vi "nanocal -- nuclear schottky fit V7.vi"() -> ()   [LabVIEW 2021] (continued)
,  \"στ1\" -> 0.000000000000   ,  \"στS\" -> 0.000000000000   ,  \"στN\" -> 0.000000000000    |>   , \n\"IDS0213_210310_RAW_cal__ref_\" ->   <|    \"ζ\" -> 0.158514180755   ,  \"τ1\" -> 0.046388884826   ,  \"τS\" -> 0.038847986012   ,  \"τN\" -> 0.058494864948   ,  \"τC\" -> 0.001325817289   ,  \"κ0\" -> 0.000000001072   ,  \"mm1\" -> 0.000176864175   ,  \"mm2\" -> 0.014706895751   ,  \"mm3\" -> 0.145604015421   ,  \"T\" -> 0.197000000000   ,  \"B\" -> 10.000000000000   ,  \"θ\" -> 0.000000000000   ,  \"Reoff\" -> 0.000000000000   ,  \"Imoff\" -> 0.000000000000   ,  \"στ1\" -> 0.000000000000   ,  \"στS\" -> 0.000000000000   ,  \"στN\" -> 0.000000000000    |>   , \n\"IDS0213_210310_RAW_cal__sam_\" ->   <|    \"ζ\" -> 0.130083148284   ,  \"τ1\" -> 0.046211117525   ,  \"τS\" -> 0.046173592526   ,  \"τN\" -> 0.081942172735   ,  \"τC\" -> 0.001380184863   ,  \"κ0\" -> 0.000000001209   ,  \"mm1\" -> 0.000155206642   ,  \"mm2\" -> 0.013836953800   ,  \"mm3\" -> 0.178380609297   ,  \"T\" -> 0.197000000000   ,  \"B\" -> 10.000000000000   ,  \"θ\" -> 0.000000000000   ,  \"Reoff\" -> 0.000000000000   ,  \"Imoff\" -> 0.000000000000   ,  \"στ1\" -> 0.000000000000   ,  \"στS\" -> 0.000000000000   ,  \"στN\" -> 0.000000000000    |>   , \n\"IDS0214_210310_RAW_cal__ref_\" ->   <|    \"ζ\" -> 0.154362032240   ,  \"τ1\" -> 0.030258273194   ,  \"τS\" -> 0.049523350330   ,  \"τN\" -> 0.040015703513   ,  \"τC\" -> 0.001328953616   ,  \"κ0\" -> 0.000000001075   ,  \"mm1\" -> 0.000174173720   ,  \"mm2\" -> 0.014698349376   ,  \"mm3\" -> 0.120075187874   ,  \"T\" -> 0.197000000000   ,  \"B\" -> 8.000000000000   ,  \"θ\" -> 0.000000000000   ,  \"Reoff\" -> 0.000000000000   ,  \"Imoff\" -> 0.000000000000   ,  \"στ1\" -> 0.000000000000   ,  \"στS\" -> 0.000000000000   ,  \"στN\" -> 0.000000000000    |>   , \n\"IDS0214_210310_RAW_cal__sam_\" ->   <|    \"ζ\" -> 0.126440702434   ,  \"τ1\" -> 0.034118036572   ,  \"τS\" -> 0.060921114440   ,  \"τN\" -> 0.059832148427   ,  \"τC\" -> 0.001404471084   ,  \"κ0\" -> 0.000000001199   ,  \"mm1\" -> 0.000154817132   ,  \"mm2\" -> 0.015271462818   ,  \"mm3\" -> 0.156117617951   ,  \"T\" -> 0.197000000000   ,  \"B\" -> 8.000000000000   ,  \"θ\" -> 0.000000000000   ,  \"Reoff\" -> 0.000000000000   ,  \"Imoff\" -> 0.000000000000   ,  \"στ1\" -> 0.000000000000   ,  \"στS\" -> 0.000000000000   ,  \"στN\" -> 0.000000000000    |>   , \n\"IDS0215_210310_RAW_cal__ref_\" ->   <|    \"ζ\" -> 0.162645417184   ,  \"τ1\" -> 0.023693851446   ,  \"τS\" -> 0.062400062170   ,  \"τN\" -> 0.026326088223   ,  \"τC\" -> 0.001322053294   ,  \"κ0\" -> 0.000000001070   ,  \"mm1\" -> 0.000182075033   ,  \"mm2\" -> 0.015525359924   ,  \"mm3\" -> 0.112465521923   ,  \"T\" -> 0.197000000000   ,  \"B\" -> 7.000000000000   ,  \"θ\" -> 0.000000000000   ,  \"Reoff\" -> 0.000000000000   ,  \"Imoff\" -> 0.000000000000   ,  \"στ1\" -> 0.000000000000   ,  \"στS\" -> 0.000000000000   ,  \"στN\" -> 0.000000000000    |>   , \n\"IDS0215_210310_RAW_cal__sam_\" ->   <|    \"ζ\" -> 0.131383255045   ,  \"τ1\" -> 0.026827335842   ,  \"τS\" -> 0.071725959535   ,  \"τN\" -> 0.047510049318   ,  \"τC\" -> 0.001407613780   ,  \"κ0\" -> 0.000000001187   ,  \"mm1\" -> 0.000160977956   ,  \"mm2\" -> 0.014932130994   ,  \"mm3\" -> 0.148043464486   ,  \"T\" -> 0.197000000000   ,  \"B\" -> 7.000000000000   ,  \"θ\" -> 0.000000000000   ,  \"Reoff\" -> 0.000000000000   ,  \"Imoff\" -> 0.000000000000   ,  \"στ1\" -> 0.000000000000   ,  \"στS\" -> 0.000000000000   ,  \"στN\" -> 0.000000000000    |>   , \n\"IDS0216_210310_RAW_cal__ref_\" ->   <|    \"ζ\" -> 0.149904026692   ,  \"τ1\" -> 0.020347243982   ,  \"τS\" -> 0.075273674904   ,  \"τN\" -> 0.020640082408   ,  \"τC\" -> 0.001432916876   ,  \"κ0\" -> 0.000000001050   ,  \"mm1\" -> 0.000184134986   ,  \"mm2\" -> 0.015328528282   ,  \"mm3\" -> 0.116559113338   ,  \"T\" -> 0.197000000000   ,  \"B\" -> 5.000000000000   ,  \"θ\" -> 0.000000000000   ,  \"Reoff\" -> 0.000000000000   ,  \"Imoff\" -> 0.000000000000   ,  \"στ1\" -> 0.000000000000   ,  \"στS\" -> 0.000000000000   ,  \"στN\" -> 0.000000000000    |>   , \n\"IDS0216_210310_RAW_cal__sam_\" ->   <|    \"ζ\" -> 0.125455081262   ,  \"τ1\" -> 0.021777951907   ,  \"τS\" -> 0.089086097551   ,  \"τN\" -> 0.033580911935   ,  \"τC\" -> 0.001437991682   ,  \"κ0\" -> 0.000000001167   ,  \"mm1\" -> 0.000158268021   ,  \"mm2\" -> 0.015150793318   ,  \"mm3\" -> 0.145963091379   ,  \"T\" -> 0.197000000000   ,  \"B\" -> 5.000000000000   ,  \"θ\" -> 0.000000000000   ,  \"Reoff\" -> 0.000000000000   ,  \"Imoff\" -> 0.000000000000   ,  \"στ1\" -> 0.000000000000   ,  \"στS\" -> 0.000000000000   ,  \"στN\" -> 0.000000000000    |>   , \n\"IDS0217_210310_RAW_cal__ref_\" ->   <|    \"ζ\" -> 0.121305227705   ,  \"τ1\" -> 0.032098202143   ,  \"τS\" -> 0.011865067519   ,  \"τN\" -> 0.005878702730   ,  \"τC\" -> 0.002147559783   ,  \"κ0\" -> 0.000000001032   ,  \"mm1\" -> 0.000202614262   ,  \"mm2\" -> 0.011552455211   ,  \"mm3\" -> 0.042386874792   ,  \"T\" -> 0.197000000000   ,  \"B\" -> 0.000000000000   ,  \"θ\" -> 0.000000000000   ,  \"Reoff\" -> 0.000000000000   ,  \"Imoff\" -> 0.000000000000   ,  \"στ1\" -> 0.000000000000   ,  \"στS\" -> 0.000000000000   ,  \"στN\" -> 0.000000000000    |>   , \n\"IDS0217_210310_RAW_cal__sam_\" ->   <|    \"ζ\" -> 0.101804363109   ,  \"τ1\" -> 0.031947692776   ,  \"τS\" -> 0.014125667853   ,  \"τN\" -> 0.006009042128   ,  \"τC\" -> 0.002323789932   ,  \"κ0\" -> 0.000000001168   ,  \"mm1\" -> 0.000188754224   ,  \"mm2\" -> 0.013103876414   ,  \"mm3\" -> 0.043163363377   ,  \"T\" -> 0.197000000000   ,  \"B\" -> 0.000000000000   ,  \"θ\" -> 0.000000000000   ,  \"Reoff\" -> 0.000000000000   ,  \"Imoff\" -> 0.000000000000   ,  \"στ1\" -> 0.000000000000   ,  \"στS\" -> 0.000000000000   ,  \"στN\" -> 0.000000000000    |>   , \n\"IDS0218_210310_RAW_cal__ref_\" ->   <|    \"ζ\" -> 0.000000000000   ,  \"τ1\" -> 0.000000000000   ,  \"τS\" -> 0.000000000000   ,  \"τN\" -> 0.000000000000   ,  \"τC\" -> 0.000000000000   ,  \"κ0\" -> 0.000000000000   ,  \"mm1\" -> 0.000000000000   ,  \"mm2\" -> 0.000000000000   ,  \"mm3\" -> 0.000000000000   ,  \"T\" -> 1.550000000000   ,  \"B\" -> 0.000000000000   ,  \"θ\" -> 0.000000000000   ,  \"Reoff\" -> 0.000000000000   ,  \"Imoff\" -> 0.000000000000   ,  \"στ1\" -> 0.000000000000   ,  \"στS\" -> 0.000000000000   ,  \"στN\" -> 0.000000000000    |>   , \n\"IDS0218_210310_RAW_cal__sam_\" ->   <|    \"ζ\" -> 0.008537038929   ,  \"τ1\" -> 0.006154643814   ,  \"τS\" -> 0.040521205127   ,  \"τN\" -> 0.000711776675   ,  \"τC\" -> 0.001925410383   ,  \"κ0\" -> 0.000000011800   ,  \"mm1\" -> 0.000015570479   ,  \"mm2\" -> 0.006036709260   ,  \"mm3\" -> 0.043612763831   ,  \"T\" -> 1.550000000000   ,  \"B\" -> 0.000000000000   ,  \"θ\" -> 0.000000000000   ,  \"Reoff\" -> -420408.163265306153   ,  \"Imoff\" -> 0.000000000000   ,  \"στ1\" -> 0.000216261088   ,  \"στS\" -> 0.000541561495   ,  \"στN\" -> 0.000022390164    |>   , \n\"IDS0219_210310_RAW_cal__ref_\" ->   <|    \"ζ\" -> 0.000000000000   ,  \"τ1\" -> 0.000000000000   ,  \"τS\" -> 0.000000000000   ,  \"τN\" -> 0.000000000000   ,  \"τC\" -> 0.000000000000   ,  \"κ0\" -> 0.000000000000   ,  \"mm1\" -> 0.000000000000   ,  \"mm2\" -> 0.000000000000   ,  \"mm3\" -> 0.000000000000   ,  \"T\" -> 1.000000000000   ,  \"B\" -> 0.000000000000   ,  \"θ\" -> 0.000000000000   ,  \"Reoff\" -> 0.000000000000   ,  \"Imoff\" -> 0.000000000000   ,  \"στ1\" -> 0.000000000000   ,  \"στS\" -> 0.000000000000   ,  \"στN\" -> 0.000000000000    |>   , \n\"IDS0219_210310_RAW_cal__sam_\" ->   <|    \"ζ\" -> 0.000000000000   ,  \"τ1\" -> 0.000000000000   ,  \"τS\" -> 0.000000000000   ,  \"τN\" -> 0.000000000000   ,  \"τC\" -> 0.000000000000   ,  \"κ0\" -> 0.000000000000   ,  \"mm1\" -> 0.000000000000   ,  \"mm2\" -> 0.000000000000   ,  \"mm3\" -> 0.000000000000   ,  \"T\" -> 1.000000000000   ,  \"B\" -> 0.000000000000   ,  \"θ\" -> 0.000000000000   ,  \"Reoff\" -> 0.000000000000   ,  \"Imoff\" -> 0.000000000000   ,  \"στ1\" -> 0.000000000000   ,  \"στS\" -> 0.000000000000   ,  \"στN\" -> 0.000000000000    |>   , \n\"IDS0220_210310_RAW_cal__ref_\" ->   <|    \"ζ\" -> 0.000000000000   ,  \"τ1\" -> 0.000000000000   ,  \"τS\" -> 0.000000000000   ,  \"τN\" -> 0.000000000000   ,  \"τC\" -> 0.000000000000   ,  \"κ0\" -> 0.000000000000   ,  \"mm1\" -> 0.000000000000   ,  \"mm2\" -> 0.000000000000   ,  \"mm3\" -> 0.000000000000   ,  \"T\" -> 0.677000000000   ,  \"B\" -> 0.000000000000   ,  \"θ\" -> 0.000000000000   ,  \"Reoff\" -> 0.000000000000   ,  \"Imoff\" -> 0.000000000000   ,  \"στ1\" -> 0.000000000000   ,  \"στS\" -> 0.000000000000   ,  \"στN\" -> 0.000000000000    |>   , \n\"IDS0220_210310_RAW_cal__sam_\" ->   <|    \"ζ\" -> 0.000000000000   ,  \"τ1\" -> 0.000000000000   ,  \"τS\" -> 0.000000000000   ,  \"τN\" -> 0.000000000000   ,  \"τC\" -> 0.000000000000   ,  \"κ0\" -> 0.000000000000   ,  \"mm1\" -> 0.000000000000   ,  \"mm2\" -> 0.000000000000   ,  \"mm3\" -> 0.000000000000   ,  \"T\" -> 0.677000000000   ,  \"B\" -> 0.000000000000   ,  \"θ\" -> 0.000000000000   ,  \"Reoff\" -> 0.000000000000   ,  \"Imoff\" -> 0.000000000000   ,  \"στ1\" -> 0.000000000000   ,  \"στS\" -> 0.000000000000   ,  \"στN\" -> 0.000000000000    |>   , \n\"IDS0224_210310_RAW_cal__ref_\" ->   <|    \"ζ\" -> 0.000000000000   ,  \"τ1\" -> 0.000000000000   ,  \"τS\" -> 0.000000000000   ,  \"τN\" -> 0.000000000000   ,  \"τC\" -> 0.000000000000   ,  \"κ0\" -> 0.000000000000   ,  \"mm1\" -> 0.000000000000   ,  \"mm2\" -> 0.000000000000   ,  \"mm3\" -> 0.000000000000   ,  \"T\" -> 0.000000000000   ,  \"B\" -> 0.000000000000   ,  \"θ\" -> 0.000000000000   ,  \"Reoff\" -> 0.000000000000   ,  \"Imoff\" -> 0.000000000000   ,  \"στ1\" -> 0.000000000000   ,  \"στS\" -> 0.000000000000   ,  \"στN\" -> 0.000000000000    |>   , \n\"IDS0224_210310_RAW_cal__sam_\" ->   <|    \"ζ\" -> 0.000000000000   ,  \"τ1\" -> 0.000000000000   ,  \"τS\" -> 0.000000000000   ,  \"τN\" -> 0.000000000000   ,  \"τC\" -> 0.000000000000   ,  \"κ0\" -> 0.000000000000   ,  \"mm1\" -> 0.000000000000   ,  \"mm2\" -> 0.000000000000   ,  \"mm3\" -> 0.000000000000   ,  \"T\" -> 0.000000000000   ,  \"B\" -> 0.000000000000   ,  \"θ\" -> 0.000000000000   ,  \"Reoff\" -> 0.000000000000   ,  \"Imoff\" -> 0.000000000000   ,  \"στ1\" -> 0.000000000000   ,  \"στS\" -> 0.000000000000   ,  \"στN\" -> 0.000000000000    |>   , \n\"IDS0293_210427_RAW_cal__ref_\" ->   <|    \"ζ\" -> 0.016384838586   ,  \"τ1\" -> 0.013784349529   ,  \"τS\" -> 0.011495286759   ,  \"τN\" -> 0.000117117954   ,  \"τC\" -> 0.004048153799   ,  \"κ0\" -> 0.000000013122   ,  \"mm1\" -> 0.000048616206   ,  \"mm2\" -> 0.013163310838   ,  \"mm3\" -> 0.016423248374   ,  \"T\" -> 1.900000000000   ,  \"B\" -> 12.000000000000   ,  \"θ\" -> 30.000000000000   ,  \"Reoff\" -> 0.000000000000   ,  \"Imoff\" -> 0.000000000000   ,  \"στ1\" -> 0.000000000000   ,  \"στS\" -> 0.000000000000   ,  \"στN\" -> 0.000000000000    |>   , \n\"IDS0293_210427_RAW_cal__sam_\" ->   <|    \"ζ\" -> 0.009769235649   ,  \"τ1\" -> 0.020538276815   ,  \"τS\" -> 0.013494754544   ,  \"τN\" -> 0.000177075548   ,  \"τC\" -> 0.005872879859   ,  \"κ0\" -> 0.000000013933   ,  \"mm1\" -> 0.000039786676   ,  \"mm2\" -> 0.018120715591   ,  \"mm3\" -> 0.022056047829   ,  \"T\" -> 1.900000000000   ,  \"B\" -> 12.000000000000   ,  \"θ\" -> 30.000000000000   ,  \"Reoff\" -> -172000.000000000000   ,  \"Imoff\" -> 0.000000000000   ,  \"στ1\" -> 0.000000000000   ,  \"στS\" -> 0.000000000000   ,  \"στN\" -> 0.000000000000    |>   , \n\"IDS0294_210427_RAW_cal__ref_\" ->   <|    \"ζ\" -> 0.017975147456   ,  \"τ1\" -> 0.015573317032   ,  \"τS\" -> 0.016697357463   ,  \"τN\" -> 0.000401487663   ,  \"τC\" -> 0.004243374884   ,  \"κ0\" -> 0.000000007622   ,  \"mm1\" -> 0.000060128790   ,  \"mm2\" -> 0.014656172673   ,  \"mm3\" -> 0.022506589842   ,  \"T\" -> 1.130000000000   ,  \"B\" -> 12.000000000000   ,  \"θ\" -> 30.000000000000   ,  \"Reoff\" -> 0.000000000000   ,  \"Imoff\" -> 0.000000000000   ,  \"στ1\" -> 0.000000000000   ,  \"στS\" -> 0.000000000000   ,  \"στN\" -> 0.000000000000    |>   , \n\"IDS0294_210427_RAW_cal__sam_\" ->   <|    \"ζ\" -> 0.010952304636   ,  \"τ1\" -> 0.020329649306   ,  \"τS\" -> 0.020621176960   ,  \"τN\" -> 0.000487558003   ,  \"τC\" -> 0.005477732780   ,  \"κ0\" -> 0.000000008194   ,  \"mm1\" -> 0.000047079068   ,  \"mm2\" -> 0.019035053021   ,  \"mm3\" -> 0.028065174256   ,  \"T\" -> 1.130000000000   ,  \"B\" -> 12.000000000000   ,  \"θ\" -> 30.000000000000   ,  \"Reoff\" -> -250000.000000000000   ,  \"Imoff\" -> 0.000000000000   ,  \"στ1\" -> 0.000000000000   ,  \"στS\" -> 0.000000000000   ,  \"στN\" -> 0.000000000000    |>   , \n\"IDS0295_210427_RAW_cal__ref_\" ->   <|    \"ζ\" -> 0.021360373560   ,  \"τ1\" -> 0.017226807214   ,  \"τS\" -> 0.021136224671   ,  \"τN\" -> 0.000857882935   ,  \"τC\" -> 0.004088468956   ,  \"κ0\" -> 0.000000005432   ,  \"mm1\" -> 0.000072090186   ,  \"mm2\" -> 0.015812919970   ,  \"mm3\" -> 0.027894175974   ,  \"T\" -> 0.830000000000   ,  \"B\" -> 12.000000000000   ,  \"θ\" -> 30.000000000000   ,  \"Reoff\" -> 0.000000000000   ,  \"Imoff\" -> 0.000000000000   ,  \"στ1\" -> 0.000000000000   ,  \"στS\" -> 0.000000000000   ,  \"στN\" -> 0.000000000000    |>   , \n\"IDS0295_210427_RAW_cal__sam_\" ->   <|    \"ζ\" -> 0.014046811833   ,  \"τ1\" -> 0.021205417259   ,  \"τS\" -> 0.025982453768   ,  \"τN\" -> 0.000985536826   ,  \"τC\" -> 0.005692013080   ,  \"κ0\" -> 0.000000005890   ,  \"mm1\" -> 0.000064969808   ,  \"mm2\" -> 0.019619534974   ,  \"mm3\" -> 0.034559730440   ,  \"T\" -> 0.830000000000   ,  \"B\" -> 12.000000000000   ,  \"θ\" -> 30.000000000000   ,  \"Reoff\" -> -401999.999999999999   ,  \"Imoff\" -> 0.000000000000   ,  \"στ1\" -> 0.000000000000   ,  \"στS\" -> 0.000000000000   ,  \"στN\" -> 0.000000000000    |>   , \n\"IDS0296_210427_RAW_cal__ref_\" ->   <|    \"ζ\" -> 0.027756025784   ,  \"τ1\" -> 0.019742757718   ,  \"τS\" -> 0.026611973171   ,  \"τN\" -> 0.001398943183   ,  \"τC\" -> 0.003482574473   ,  \"κ0\" -> 0.000000003907   ,  \"mm1\" -> 0.000083653758   ,  \"mm2\" -> 0.017774350196   ,  \"mm3\" -> 0.034155716307   ,  \"T\" -> 0.620000000000   ,  \"B\" -> 12.000000000000   ,  \"θ\" -> 30.000000000000   ,  \"Reoff\" -> 0.000000000000   ,  \"Imoff\" -> 0.000000000000   ,  \"στ1\" -> 0.000000000000   ,  \"στS\" -> 0.000000000000   ,  \"στN\" -> 0.000000000000    |>   , \n\"IDS0296_210427_RAW_cal__sam_\" ->   <|    \"ζ\" -> 0.017388662959   ,  \"τ1\" -> 0.016835863979   ,  \"τS\" -> 0.033051741689   ,  \"τN\" -> 0.001876583642   ,  \"τC\" -> 0.004718731610   ,  \"κ0\" -> 0.000000004257   ,  \"mm1\" -> 0.000070854167   ,  \"mm2\" -> 0.015532685015   ,  \"mm3\" -> 0.041486738616   ,  \"T\" -> 0.620000000000   ,  \"B\" -> 12.000000000000   ,  \"θ\" -> 30.000000000000   ,  \"Reoff\" -> -602409.638554215430   ,  \"Imoff\" -> 0.000000000000   ,  \"στ1\" -> 0.000000000000   ,  \"στS\" -> 0.000000000000   ,  \"στN\" -> 0.000000000000    |>   , \n\"IDS0297_210427_RAW_cal__ref_\" ->   <|    \"ζ\" -> 0.034775017342   ,  \"τ1\" -> 0.018923965005   ,  \"τS\" -> 0.030086686370   ,  \"τN\" -> 0.002286572055   ,  \"τC\" -> 0.002714831651   ,  \"κ0\" -> 0.000000003294   ,  \"mm1\" -> 0.000084124720   ,  \"mm2\" -> 0.016628755460   ,  \"mm3\" -> 0.038424955523   ,  \"T\" -> 0.530000000000   ,  \"B\" -> 12.000000000000   ,  \"θ\" -> 30.000000000000   ,  \"Reoff\" -> 0.000000000000   ,  \"Imoff\" -> 0.000000000000   ,  \"στ1\" -> 0.000000000000   ,  \"στS\" -> 0.000000000000   ,  \"στN\" -> 0.000000000000    |>   , \n\"IDS0297_210427_RAW_cal__sam_\" ->   <|    \"ζ\" -> 0.020542184284   ,  \"τ1\" -> 0.020760439172   ,  \"τS\" -> 0.037341907366   ,  \"τN\" -> 0.003219016214   ,  \"τC\" -> 0.004292471555   ,  \"κ0\" -> 0.000000003557   ,  \"mm1\" -> 0.000077795275   ,  \"mm2\" -> 0.018267084885   ,  \"mm3\" -> 0.048102164115   ,  \"T\" -> 0.530000000000   ,  \"B\" -> 12.000000000000   ,  \"θ\" -> 30.000000000000   ,  \"Reoff\" -> -602409.638554215430   ,  \"Imoff\" -> 0.000000000000   ,  \"στ1\" -> 0.000000000000   ,  \"στS\" -> 0.000000000000   ,  \"στN\" -> 0.000000000000    |>   , \n\"IDS0298_210427_RAW_cal__ref_\" ->   <|    \"ζ\" -> 0.046440102993   ,  \"τ1\" -> 0.018907201785   ,  \"τS\" -> 0.034021724611   ,  \"τN\" -> 0.004470088018   ,  \"τC\" -> 0.002281608431   ,  \"κ0\" -> 0.000000002638   ,  \"mm1\" -> 0.000095393981   ,  \"mm2\" -> 0.015614445786   ,  \"mm3\" -> 0.045758346821   ,  \"T\" -> 0.430000000000   ,  \"B\" -> 12.000000000000   ,  \"θ\" -> 30.000000000000   ,  \"Reoff\" -> -3126506.024096369740   ,  \"Imoff\" -> 0.000000000000   ,  \"στ1\" -> 0.013462619776   ,  \"στS\" -> 0.001228313505   ,  \"στN\" -> 0.000000000000    |>   , \n\"IDS0298_210427_RAW_cal__sam_\" ->   <|    \"ζ\" -> 0.028504600675   ,  \"τ1\" -> 0.017787596977   ,  \"τS\" -> 0.043231501144   ,  \"τN\" -> 0.005920795525   ,  \"τC\" -> 0.002978583592   ,  \"κ0\" -> 0.000000002855   ,  \"mm1\" -> 0.000077491236   ,  \"mm2\" -> 0.014973532625   ,  \"mm3\" -> 0.056268519966   ,  \"T\" -> 0.430000000000   ,  \"B\" -> 12.000000000000   ,  \"θ\" -> 30.000000000000   ,  \"Reoff\" -> -2300000.000000000000   ,  \"Imoff\" -> 0.000000000000   ,  \"στ1\" -> 0.000000000000   ,  \"στS\" -> 0.000000000000   ,  \"στN\" -> 0.000000000000    |>   , \n\"IDS0299_210427_RAW_cal__ref_\" ->   <|    \"ζ\" -> 0.060451978173   ,  \"τ1\" -> 0.020932044867   ,  \"τS\" -> 0.038339527687   ,  \"τN\" -> 0.009019484504   ,  \"τC\" -> 0.001991911381   ,  \"κ0\" -> 0.000000002121   ,  \"mm1\" -> 0.000108517518   ,  \"mm2\" -> 0.015468645240   ,  \"mm3\" -> 0.057568751652   ,  \"T\" -> 0.360000000000   ,  \"B\" -> 12.000000000000   ,  \"θ\" -> 30.000000000000   ,  \"Reoff\" -> -4033132.530120491980   ,  \"Imoff\" -> 0.000000000000   ,  \"στ1\" -> 0.008893690340   ,  \"στS\" -> 0.001445462224   ,  \"στN\" -> 0.000000000000    |>   , \n\"IDS0299_210427_RAW_cal__sam_\" ->   <|    \"ζ\" -> 0.036443500348   ,  \"τ1\" -> 0.020154057220   ,  \"τS\" -> 0.048932682096   ,  \"τN\" -> 0.011280238135   ,  \"τC\" -> 0.002753749788   ,  \"κ0\" -> 0.000000002299   ,  \"mm1\" -> 0.000091994249   ,  \"mm2\" -> 0.015410264614   ,  \"mm3\" -> 0.069812837955   ,  \"T\" -> 0.360000000000   ,  \"B\" -> 12.000000000000   ,  \"θ\" -> 30.000000000000   ,  \"Reoff\" -> -2590361.445783123380   ,  \"Imoff\" -> 0.000000000000   ,  \"στ1\" -> 0.000000000000   ,  \"στS\" -> 0.000000000000   ,  \"στN\" -> 0.000000000000    |>   , \n\"IDS0300_210427_RAW_cal__ref_\" ->   <|    \"ζ\" -> 0.339239140566   ,  \"τ1\" -> 0.049004480747   ,  \"τS\" -> 0.154731734875   ,  \"τN\" -> 0.405076937535   ,  \"τC\" -> 0.001214632941   ,  \"κ0\" -> 0.000000000422   ,  \"mm1\" -> 0.000306310339   ,  \"mm2\" -> 0.012966272526   ,  \"mm3\" -> 0.786664216144   ,  \"T\" -> 0.140000000000   ,  \"B\" -> 12.000000000000   ,  \"θ\" -> 30.000000000000   ,  \"Reoff\" -> -103762048.192771077000   ,  \"Imoff\" -> 0.000000000000   ,  \"στ1\" -> 0.015510670555   ,  \"στS\" -> 0.015380063166   ,  \"στN\" -> 0.000000000000    |>   , \n\"IDS0300_210427_RAW_cal__sam_\" ->   <|    \"ζ\" -> 0.180438460866   ,  \"τ1\" -> 0.048255220427   ,  \"τS\" -> 0.195496614309   ,  \"τN\" -> 0.254134303670   ,  \"τC\" -> 0.001384159230   ,  \"κ0\" -> 0.000000000598   ,  \"mm1\" -> 0.000210501936   ,  \"mm2\" -> 0.019979803647   ,  \"mm3\" -> 0.560210702851   ,  \"T\" -> 0.140000000000   ,  \"B\" -> 12.000000000000   ,  \"θ\" -> 30.000000000000   ,  \"Reoff\" -> -29759036.144578307900   ,  \"Imoff\" -> 0.000000000000   ,  \"στ1\" -> 0.000000000000   ,  \"στS\" -> 0.000000000000   ,  \"στN\" -> 0.000000000000    |>   , \n\"IDS0301_210831_RAW_cal__ref_\" ->   <|    \"ζ\" -> 0.083102815664   ,  \"τ1\" -> 0.023587336655   ,  \"τS\" -> 0.043380203208   ,  \"τN\" -> 0.014582503470   ,  \"τC\" -> 0.001563516475   ,  \"κ0\" -> 0.000000001737   ,  \"mm1\" -> 0.000116373060   ,  \"mm2\" -> 0.015882403600   ,  \"mm3\" -> 0.071931647277   ,  \"T\" -> 0.300000000000   ,  \"B\" -> 12.000000000000   ,  \"θ\" -> 30.000000000000   ,  \"Reoff\" -> -7370481.927710846070   ,  \"Imoff\" -> 0.000000000000   ,  \"στ1\" -> 0.008245172960   ,  \"στS\" -> 0.001836119711   ,  \"στN\" -> 0.000000000000    |>   , \n\"IDS0301_210831_RAW_cal__sam_\" ->   <|    \"ζ\" -> 0.050368719514   ,  \"τ1\" -> 0.024372679774   ,  \"τS\" -> 0.056652990002   ,  \"τN\" -> 0.018868210601   ,  \"τC\" -> 0.002169557672   ,  \"κ0\" -> 0.000000001890   ,  \"mm1\" -> 0.000100537132   ,  \"mm2\" -> 0.016885854065   ,  \"mm3\" -> 0.088880953022   ,  \"T\" -> 0.300000000000   ,  \"B\" -> 12.000000000000   ,  \"θ\" -> 30.000000000000   ,  \"Reoff\" -> -5240963.855421677230   ,  \"Imoff\" -> 0.000000000000   ,  \"στ1\" -> 0.000000000000   ,  \"στS\" -> 0.000000000000   ,  \"στN\" -> 0.000000000000    |>   , \n\"IDS0302_210831_RAW_cal__ref_\" ->   <|    \"ζ\" -> 0.118276511674   ,  \"τ1\" -> 0.024667236768   ,  \"τS\" -> 0.048709348590   ,  \"τN\" -> 0.031529020299   ,  \"τC\" -> 0.001279390112   ,  \"κ0\" -> 0.000000001362   ,  \"mm1\" -> 0.000132517053   ,  \"mm2\" -> 0.013437351030   ,  \"mm3\" -> 0.102105442061   ,  \"T\" -> 0.250000000000   ,  \"B\" -> 12.000000000000   ,  \"θ\" -> 30.000000000000   ,  \"Reoff\" -> -14030120.481927707800   ,  \"Imoff\" -> 0.000000000000   ,  \"στ1\" -> 0.005527591080   ,  \"στS\" -> 0.002366766012   ,  \"στN\" -> 0.000000000000    |>   , \n\"IDS0302_210831_RAW_cal__sam_\" ->   <|    \"ζ\" -> 0.070275268573   ,  \"τ1\" -> 0.028026457127   ,  \"τS\" -> 0.065297867120   ,  \"τN\" -> 0.040008645873   ,  \"τC\" -> 0.001817885465   ,  \"κ0\" -> 0.000000001504   ,  \"mm1\" -> 0.000116520135   ,  \"mm2\" -> 0.015851021970   ,  \"mm3\" -> 0.126583756963   ,  \"T\" -> 0.250000000000   ,  \"B\" -> 12.000000000000   ,  \"θ\" -> 30.000000000000   ,  \"Reoff\" -> -8554216.867469877010   ,  \"Imoff\" -> 0.000000000000   ,  \"στ1\" -> 0.000000000000   ,  \"στS\" -> 0.000000000000   ,  \"στN\" -> 0.000000000000    |>   , \n\"IDS0303_210831_RAW_cal__ref_\" ->   <|    \"ζ\" -> 0.210201005272   ,  \"τ1\" -> 0.036306230706   ,  \"τS\" -> 0.066320996268   ,  \"τN\" -> 0.080911010033   ,  \"τC\" -> 0.001077377701   ,  \"κ0\" -> 0.000000001046   ,  \"mm1\" -> 0.000185060428   ,  \"mm2\" -> 0.014681839337   ,  \"mm3\" -> 0.200697030676   ,  \"T\" -> 0.200000000000   ,  \"B\" -> 12.000000000000   ,  \"θ\" -> 30.000000000000   ,  \"Reoff\" -> -29165662.650602400300   ,  \"Imoff\" -> 0.000000000000   ,  \"στ1\" -> 0.007631270383   ,  \"στS\" -> 0.005042040043   ,  \"στN\" -> 0.000000000000    |>   , \n\"IDS0303_210831_RAW_cal__sam_\" ->   <|    \"ζ\" -> 0.127771364483   ,  \"τ1\" -> 0.034431916362   ,  \"τS\" -> 0.086066228156   ,  \"τN\" -> 0.103317216156   ,  \"τC\" -> 0.001469970272   ,  \"κ0\" -> 0.000000001169   ,  \"mm1\" -> 0.000164317810   ,  \"mm2\" -> 0.014420189715   ,  \"mm3\" -> 0.234898604511   ,  \"T\" -> 0.200000000000   ,  \"B\" -> 12.000000000000   ,  \"θ\" -> 30.000000000000   ,  \"Reoff\" -> -17831325.301204815500   ,  \"Imoff\" -> 0.000000000000   ,  \"στ1\" -> 0.000000000000   ,  \"στS\" -> 0.000000000000   ,  \"στN\" -> 0.000000000000    |>   , \n\"IDS0304_210831_RAW_cal__ref_\" ->   <|    \"ζ\" -> 0.269991588498   ,  \"τ1\" -> 0.042008612133   ,  \"τS\" -> 0.092789631538   ,  \"τN\" -> 0.170188261604   ,  \"τC\" -> 0.001076825929   ,  \"κ0\" -> 0.000000000745   ,  \"mm1\" -> 0.000227270912   ,  \"mm2\" -> 0.013732742400   ,  \"mm3\" -> 0.363105137001   ,  \"T\" -> 0.170000000000   ,  \"B\" -> 12.000000000000   ,  \"θ\" -> 30.000000000000   ,  \"Reoff\" -> -52171686.746987946300   ,  \"Imoff\" -> 0.000000000000   ,  \"στ1\" -> 0.010619336598   ,  \"στS\" -> 0.010896322396   ,  \"στN\" -> 0.000000000000    |>   , \n\"IDS0304_210831_RAW_cal__sam_\" ->   <|    \"ζ\" -> 0.166070461716   ,  \"τ1\" -> 0.041003941798   ,  \"τS\" -> 0.114733330952   ,  \"τN\" -> 0.164402286708   ,  \"τC\" -> 0.001371627013   ,  \"κ0\" -> 0.000000000890   ,  \"mm1\" -> 0.000193629021   ,  \"mm2\" -> 0.015725118152   ,  \"mm3\" -> 0.351948620204   ,  \"T\" -> 0.170000000000   ,  \"B\" -> 12.000000000000   ,  \"θ\" -> 30.000000000000   ,  \"Reoff\" -> -32409638.554216861700   ,  \"Imoff\" -> 0.000000000000   ,  \"στ1\" -> 0.000000000000   ,  \"στS\" -> 0.000000000000   ,  \"στN\" -> 0.000000000000    |>   , \n\"IDS0305_210831_RAW_cal__ref_\" ->   <|    \"ζ\" -> 0.281505704242   ,  \"τ1\" -> 0.044410384222   ,  \"τS\" -> 0.104666316175   ,  \"τN\" -> 0.238180601074   ,  \"τC\" -> 0.001077670144   ,  \"κ0\" -> 0.000000000630   ,  \"mm1\" -> 0.000235234007   ,  \"mm2\" -> 0.012702965231   ,  \"mm3\" -> 0.471910135265   ,  \"T\" -> 0.160000000000   ,  \"B\" -> 12.000000000000   ,  \"θ\" -> 30.000000000000   ,  \"Reoff\" -> -64885542.168674700000   ,  \"Imoff\" -> 0.000000000000   ,  \"στ1\" -> 0.013415612751   ,  \"στS\" -> 0.014884617591   ,  \"στN\" -> 0.000000000000    |>   , \n\"IDS0305_210831_RAW_cal__sam_\" ->   <|    \"ζ\" -> 0.168984978681   ,  \"τ1\" -> 0.042944879888   ,  \"τS\" -> 0.137797235983   ,  \"τN\" -> 0.201278537585   ,  \"τC\" -> 0.001423239236   ,  \"κ0\" -> 0.000000000771   ,  \"mm1\" -> 0.000204183123   ,  \"mm2\" -> 0.016435652766   ,  \"mm3\" -> 0.424102769171   ,  \"T\" -> 0.160000000000   ,  \"B\" -> 12.000000000000   ,  \"θ\" -> 30.000000000000   ,  \"Reoff\" -> -36385542.168674692500   ,  \"Imoff\" -> 0.000000000000   ,  \"στ1\" -> 0.000000000000   ,  \"στS\" -> 0.000000000000   ,  \"στN\" -> 0.000000000000    |>   , \n\"IDS0306_210831_RAW_cal__ref_\" ->   <|    \"ζ\" -> 0.013593052641   ,  \"τ1\" -> 0.010989385662   ,  \"τS\" -> 0.007947176041   ,  \"τN\" -> 0.000037757079   ,  \"τC\" -> 0.003572854733   ,  \"κ0\" -> 0.000000023548   ,  \"mm1\" -> 0.000033287498   ,  \"mm2\" -> 0.010587625602   ,  \"mm3\" -> 0.012034800032   ,  \"T\" -> 3.100000000000   ,  \"B\" -> 12.000000000000   ,  \"θ\" -> 30.000000000000   ,  \"Reoff\" -> 0.000000000000   ,  \"Imoff\" -> 0.000000000000   ,  \"στ1\" -> 0.000000000000   ,  \"στS\" -> 0.000000000000   ,  \"στN\" -> 0.000000000000    |>   , \n\"IDS0306_210831_RAW_cal__sam_\" ->   <|    \"ζ\" -> 0.007685785961   ,  \"τ1\" -> 0.018036205476   ,  \"τS\" -> 0.008821186550   ,  \"τN\" -> 0.000090733660   ,  \"τC\" -> 0.005794291982   ,  \"κ0\" -> 0.000000024405   ,  \"mm1\" -> 0.000026803010   ,  \"mm2\" -> 0.014306219949   ,  \"mm3\" -> 0.018477889820   ,  \"T\" -> 3.100000000000   ,  \"B\" -> 12.000000000000   ,  \"θ\" -> 30.000000000000   ,  \"Reoff\" -> -62000.000000000000   ,  \"Imoff\" -> 0.000000000000   ,  \"στ1\" -> 0.000000000000   ,  \"στS\" -> 0.000000000000   ,  \"στN\" -> 0.000000000000    |>   , \n\"IDS0310_210901_RAW_cal__ref_\" ->   <|    \"ζ\" -> 0.294196069585   ,  \"τ1\" -> 0.054258754823   ,  \"τS\" -> 0.066187792705   ,  \"τN\" -> 0.210307390595   ,  \"τC\" -> 0.001028009628   ,  \"κ0\" -> 0.000000000624   ,  \"mm1\" -> 0.000231504342   ,  \"mm2\" -> 0.011693954387   ,  \"mm3\" -> 0.401200285208   ,  \"T\" -> 0.157000000000   ,  \"B\" -> 12.000000000000   ,  \"θ\" -> 45.000000000000   ,  \"Reoff\" -> -66590361.445783138300   ,  \"Imoff\" -> 0.000000000000   ,  \"στ1\" -> 0.021984252892   ,  \"στS\" -> 0.027799498625   ,  \"στN\" -> 0.000000000000    |>   , \n\"IDS0310_210901_RAW_cal__sam_\" ->   <|    \"ζ\" -> 0.295520923520   ,  \"τ1\" -> 0.054772440405   ,  \"τS\" -> 0.071814005451   ,  \"τN\" -> 0.249593767169   ,  \"τC\" -> 0.001103632155   ,  \"κ0\" -> 0.000000000625   ,  \"mm1\" -> 0.000249422174   ,  \"mm2\" -> 0.011160480416   ,  \"mm3\" -> 0.460856664381   ,  \"T\" -> 0.157000000000   ,  \"B\" -> 12.000000000000   ,  \"θ\" -> 45.000000000000   ,  \"Reoff\" -> 0.000000000000   ,  \"Imoff\" -> 0.000000000000   ,  \"στ1\" -> 0.000000000000   ,  \"στS\" -> 0.000000000000   ,  \"στN\" -> 0.000000000000    |>   , \n\"IDS0311_210901_RAW_cal__ref_\" ->   <|    \"ζ\" -> 0.508858563878   ,  \"τ1\" -> 0.072484057695   ,  \"τS\" -> 0.091005153910   ,  \"τN\" -> 0.493200178379   ,  \"τC\" -> 0.000985068264   ,  \"κ0\" -> 0.000000000428   ,  \"mm1\" -> 0.000330595844   ,  \"mm2\" -> 0.010594734788   ,  \"mm3\" -> 0.944027014014   ,  \"T\" -> 0.120000000000   ,  \"B\" -> 12.000000000000   ,  \"θ\" -> 45.000000000000   ,  \"Reoff\" -> -111015060.240963846000   ,  \"Imoff\" -> 0.000000000000   ,  \"στ1\" -> 0.030760368517   ,  \"στS\" -> 0.002434782882   ,  \"στN\" -> 0.000000000000    |>   , \n\"IDS0311_210901_RAW_cal__sam_\" ->   <|    \"ζ\" -> 0.523545279740   ,  \"τ1\" -> 0.065613539167   ,  \"τS\" -> 0.100000000000   ,  \"τN\" -> 0.424083114177   ,  \"τC\" -> 0.000911255863   ,  \"κ0\" -> 0.000000000418   ,  \"mm1\" -> 0.000311888140   ,  \"mm2\" -> 0.011767552098   ,  \"mm3\" -> 0.852909709588   ,  \"T\" -> 0.120000000000   ,  \"B\" -> 12.000000000000   ,  \"θ\" -> 45.000000000000   ,  \"Reoff\" -> 0.000000000000   ,  \"Imoff\" -> 0.000000000000   ,  \"στ1\" -> 0.000000000000   ,  \"στS\" -> 0.000000000000   ,  \"στN\" -> 0.000000000000    |>   , \n\"IDS0312_210901_RAW_cal__ref_\" ->   <|    \"ζ\" -> 0.259527657087   ,  \"τ1\" -> 0.050950801212   ,  \"τS\" -> 0.056257064354   ,  \"τN\" -> 0.162412214705   ,  \"τC\" -> 0.001029454962   ,  \"κ0\" -> 0.000000000750   ,  \"mm1\" -> 0.000209665786   ,  \"mm2\" -> 0.011572567257   ,  \"mm3\" -> 0.315618027862   ,  \"T\" -> 0.170000000000   ,  \"B\" -> 12.000000000000   ,  \"θ\" -> 45.000000000000   ,  \"Reoff\" -> -47551204.819277107700   ,  \"Imoff\" -> 0.000000000000   ,  \"στ1\" -> 0.007568346917   ,  \"στS\" -> 0.006727038440   ,  \"στN\" -> 0.000000000000    |>   , \n\"IDS0312_210901_RAW_cal__sam_\" ->   <|    \"ζ\" -> 0.273742116471   ,  \"τ1\" -> 0.052262909995   ,  \"τS\" -> 0.060554036646   ,  \"τN\" -> 0.154269705680   ,  \"τC\" -> 0.001074144337   ,  \"κ0\" -> 0.000000000753   ,  \"mm1\" -> 0.000228314156   ,  \"mm2\" -> 0.012990527394   ,  \"mm3\" -> 0.313748261000   ,  \"T\" -> 0.170000000000   ,  \"B\" -> 12.000000000000   ,  \"θ\" -> 45.000000000000   ,  \"Reoff\" -> 0.000000000000   ,  \"Imoff\" -> 0.000000000000   ,  \"στ1\" -> 0.000000000000   ,  \"στS\" -> 0.000000000000   ,  \"στN\" -> 0.000000000000    |>   , \n\"IDS0313_210901_RAW_cal__ref_\" ->   <|    \"ζ\" -> 0.214632480491   ,  \"τ1\" -> 0.045379665546   ,  \"τS\" -> 0.046142273352   ,  \"τN\" -> 0.090406420650   ,  \"τC\" -> 0.001068824468   ,  \"κ0\" -> 0.000000001040   ,  \"mm1\" -> 0.000185914799   ,  \"mm2\" -> 0.012974151189   ,  \"mm3\" -> 0.199144902930   ,  \"T\" -> 0.200000000000   ,  \"B\" -> 12.000000000000   ,  \"θ\" -> 45.000000000000   ,  \"Reoff\" -> -30325301.204819276900   ,  \"Imoff\" -> 0.000000000000   ,  \"στ1\" -> 0.006255922124   ,  \"στS\" -> 0.003795789504   ,  \"στN\" -> 0.000000000000    |>   , \n\"IDS0313_210901_RAW_cal__sam_\" ->   <|    \"ζ\" -> 0.215688135788   ,  \"τ1\" -> 0.043710888546   ,  \"τS\" -> 0.044756474141   ,  \"τN\" -> 0.090222547904   ,  \"τC\" -> 0.001049781785   ,  \"κ0\" -> 0.000000001047   ,  \"mm1\" -> 0.000183308759   ,  \"mm2\" -> 0.012306282012   ,  \"mm3\" -> 0.196363475241   ,  \"T\" -> 0.200000000000   ,  \"B\" -> 12.000000000000   ,  \"θ\" -> 45.000000000000   ,  \"Reoff\" -> 0.000000000000   ,  \"Imoff\" -> 0.000000000000   ,  \"στ1\" -> 0.000000000000   ,  \"στS\" -> 0.000000000000   ,  \"στN\" -> 0.000000000000    |>   , \n\"IDS0314_210901_RAW_cal__ref_\" ->   <|    \"ζ\" -> 0.122092266901   ,  \"τ1\" -> 0.034197829393   ,  \"τS\" -> 0.036704742397   ,  \"τN\" -> 0.033844850691   ,  \"τC\" -> 0.001292192977   ,  \"κ0\" -> 0.000000001353   ,  \"mm1\" -> 0.000136749869   ,  \"mm2\" -> 0.014475424463   ,  \"mm3\" -> 0.100041000875   ,  \"T\" -> 0.255000000000   ,  \"B\" -> 12.000000000000   ,  \"θ\" -> 45.000000000000   ,  \"Reoff\" -> -14006024.096385538600   ,  \"Imoff\" -> 0.000000000000   ,  \"στ1\" -> 0.005419306546   ,  \"στS\" -> 0.001902499220   ,  \"στN\" -> 0.000000000000    |>   , \n\"IDS0314_210901_RAW_cal__sam_\" ->   <|    \"ζ\" -> 0.118583992968   ,  \"τ1\" -> 0.035232851003   ,  \"τS\" -> 0.037458022816   ,  \"τN\" -> 0.033724509363   ,  \"τC\" -> 0.001440922263   ,  \"κ0\" -> 0.000000001360   ,  \"mm1\" -> 0.000148167008   ,  \"mm2\" -> 0.015055022209   ,  \"mm3\" -> 0.101094225124   ,  \"T\" -> 0.255000000000   ,  \"B\" -> 12.000000000000   ,  \"θ\" -> 45.000000000000   ,  \"Reoff\" -> 0.000000000000   ,  \"Imoff\" -> 0.000000000000   ,  \"στ1\" -> 0.000000000000   ,  \"στS\" -> 0.000000000000   ,  \"στN\" -> 0.000000000000    |>   , \n\"IDS0315_210901_RAW_cal__ref_\" ->   <|    \"ζ\" -> 0.083764042578   ,  \"τ1\" -> 0.028404690940   ,  \"τS\" -> 0.032596022406   ,  \"τN\" -> 0.016694646015   ,  \"τC\" -> 0.001528847398   ,  \"κ0\" -> 0.000000001734   ,  \"mm1\" -> 0.000113603931   ,  \"mm2\" -> 0.015380769719   ,  \"mm3\" -> 0.067858618758   ,  \"T\" -> 0.300000000000   ,  \"B\" -> 12.000000000000   ,  \"θ\" -> 45.000000000000   ,  \"Reoff\" -> -7659638.554216861730   ,  \"Imoff\" -> 0.000000000000   ,  \"στ1\" -> 0.006630999900   ,  \"στS\" -> 0.001474626278   ,  \"στN\" -> 0.000000000000    |>   , \n\"IDS0315_210901_RAW_cal__sam_\" ->   <|    \"ζ\" -> 0.085152769414   ,  \"τ1\" -> 0.029001116263   ,  \"τS\" -> 0.032604663993   ,  \"τN\" -> 0.016878763935   ,  \"τC\" -> 0.001443524845   ,  \"κ0\" -> 0.000000001728   ,  \"mm1\" -> 0.000109149910   ,  \"mm2\" -> 0.015549242931   ,  \"mm3\" -> 0.068483327123   ,  \"T\" -> 0.300000000000   ,  \"B\" -> 12.000000000000   ,  \"θ\" -> 45.000000000000   ,  \"Reoff\" -> 0.000000000000   ,  \"Imoff\" -> 0.000000000000   ,  \"στ1\" -> 0.000000000000   ,  \"στS\" -> 0.000000000000   ,  \"στN\" -> 0.000000000000    |>   , \n\"IDS0316_210901_RAW_cal__ref_\" ->   <|    \"ζ\" -> 0.059431977734   ,  \"τ1\" -> 0.025344964439   ,  \"τS\" -> 0.030187831822   ,  \"τN\" -> 0.009997229668   ,  \"τC\" -> 0.001837989117   ,  \"κ0\" -> 0.000000002120   ,  \"mm1\" -> 0.000097780180   ,  \"mm2\" -> 0.015899559471   ,  \"mm3\" -> 0.053758953075   ,  \"T\" -> 0.360000000000   ,  \"B\" -> 12.000000000000   ,  \"θ\" -> 45.000000000000   ,  \"Reoff\" -> -3126506.024096369740   ,  \"Imoff\" -> 0.000000000000   ,  \"στ1\" -> 0.002854320609   ,  \"στS\" -> 0.000336853437   ,  \"στN\" -> 0.000497959558    |>   , \n\"IDS0316_210901_RAW_cal__sam_\" ->   <|    \"ζ\" -> 0.061011838044   ,  \"τ1\" -> 0.025440548989   ,  \"τS\" -> 0.030028053978   ,  \"τN\" -> 0.010140731955   ,  \"τC\" -> 0.001895079687   ,  \"κ0\" -> 0.000000002115   ,  \"mm1\" -> 0.000103163383   ,  \"mm2\" -> 0.015856737579   ,  \"mm3\" -> 0.053995285109   ,  \"T\" -> 0.360000000000   ,  \"B\" -> 12.000000000000   ,  \"θ\" -> 45.000000000000   ,  \"Reoff\" -> 0.000000000000   ,  \"Imoff\" -> 0.000000000000   ,  \"στ1\" -> 0.000000000000   ,  \"στS\" -> 0.000000000000   ,  \"στN\" -> 0.000000000000    |>   , \n\"IDS0317_210901_RAW_cal__ref_\" ->   <|    \"ζ\" -> 0.044144689760   ,  \"τ1\" -> 0.021030727933   ,  \"τS\" -> 0.027802850368   ,  \"τN\" -> 0.005306153044   ,  \"τC\" -> 0.002039269513   ,  \"κ0\" -> 0.000000002643   ,  \"mm1\" -> 0.000080764182   ,  \"mm2\" -> 0.015493151772   ,  \"mm3\" -> 0.042066671588   ,  \"T\" -> 0.430000000000   ,  \"B\" -> 12.000000000000   ,  \"θ\" -> 45.000000000000   ,  \"Reoff\" -> -2219879.518072277310   ,  \"Imoff\" -> 0.000000000000   ,  \"στ1\" -> 0.001811234684   ,  \"στS\" -> 0.000219110470   ,  \"στN\" -> 0.000329233021    |>   , \n\"IDS0317_210901_RAW_cal__sam_\" ->   <|    \"ζ\" -> 0.046686299518   ,  \"τ1\" -> 0.021011215626   ,  \"τS\" -> 0.027633142317   ,  \"τN\" -> 0.005348477555   ,  \"τC\" -> 0.002098477650   ,  \"κ0\" -> 0.000000002635   ,  \"mm1\" -> 0.000087510938   ,  \"mm2\" -> 0.015436995488   ,  \"mm3\" -> 0.042106596506   ,  \"T\" -> 0.430000000000   ,  \"B\" -> 12.000000000000   ,  \"θ\" -> 45.000000000000   ,  \"Reoff\" -> 0.000000000000   ,  \"Imoff\" -> 0.000000000000   ,  \"στ1\" -> 0.000000000000   ,  \"στS\" -> 0.000000000000   ,  \"στN\" -> 0.000000000000    |>   , \n\"IDS0318_210901_RAW_cal__ref_\" ->   <|    \"ζ\" -> 0.032848823108   ,  \"τ1\" -> 0.018119264501   ,  \"τS\" -> 0.025633128962   ,  \"τN\" -> 0.002741342485   ,  \"τC\" -> 0.002539258002   ,  \"κ0\" -> 0.000000003301   ,  \"mm1\" -> 0.000073876379   ,  \"mm2\" -> 0.015052062662   ,  \"mm3\" -> 0.034839122902   ,  \"T\" -> 0.530000000000   ,  \"B\" -> 12.000000000000   ,  \"θ\" -> 45.000000000000   ,  \"Reoff\" -> -1020408.163265287880   ,  \"Imoff\" -> 0.000000000000   ,  \"στ1\" -> 0.000541293278   ,  \"στS\" -> 0.000098746270   ,  \"στN\" -> 0.000060245222    |>   , \n\"IDS0318_210901_RAW_cal__sam_\" ->   <|    \"ζ\" -> 0.035204330012   ,  \"τ1\" -> 0.021011523093   ,  \"τS\" -> 0.025247316079   ,  \"τN\" -> 0.002718647875   ,  \"τC\" -> 0.003091727575   ,  \"κ0\" -> 0.000000003296   ,  \"mm1\" -> 0.000094318646   ,  \"mm2\" -> 0.017045496493   ,  \"mm3\" -> 0.035913922507   ,  \"T\" -> 0.530000000000   ,  \"B\" -> 12.000000000000   ,  \"θ\" -> 45.000000000000   ,  \"Reoff\" -> 0.000000000000   ,  \"Imoff\" -> 0.000000000000   ,  \"στ1\" -> 0.000000000000   ,  \"στS\" -> 0.000000000000   ,  \"στN\" -> 0.000000000000    |>   , \n\"IDS0319_210901_RAW_cal__ref_\" ->   <|    \"ζ\" -> 0.027000577828   ,  \"τ1\" -> 0.015965757563   ,  \"τS\" -> 0.024178947820   ,  \"τN\" -> 0.001643909719   ,  \"τC\" -> 0.002756663641   ,  \"κ0\" -> 0.000000003916   ,  \"mm1\" -> 0.000065386105   ,  \"mm2\" -> 0.014174024052   ,  \"mm3\" -> 0.031003100660   ,  \"T\" -> 0.620000000000   ,  \"B\" -> 12.000000000000   ,  \"θ\" -> 45.000000000000   ,  \"Reoff\" -> -897959.183673471211   ,  \"Imoff\" -> 0.000000000000   ,  \"στ1\" -> 0.001366735368   ,  \"στS\" -> 0.000249386446   ,  \"στN\" -> 0.000075862770    |>   , \n\"IDS0319_210901_RAW_cal__sam_\" ->   <|    \"ζ\" -> 0.030862035723   ,  \"τ1\" -> 0.019328530751   ,  \"τS\" -> 0.023568572597   ,  \"τN\" -> 0.001701966614   ,  \"τC\" -> 0.003453790534   ,  \"κ0\" -> 0.000000003906   ,  \"mm1\" -> 0.000090824021   ,  \"mm2\" -> 0.016669294779   ,  \"mm3\" -> 0.032072641980   ,  \"T\" -> 0.620000000000   ,  \"B\" -> 12.000000000000   ,  \"θ\" -> 45.000000000000   ,  \"Reoff\" -> 0.000000000000   ,  \"Imoff\" -> 0.000000000000   ,  \"στ1\" -> 0.000000000000   ,  \"στS\" -> 0.000000000000   ,  \"στN\" -> 0.000000000000    |>   , \n\"IDS0320_210901_RAW_cal__ref_\" ->   <|    \"ζ\" -> 0.020582548855   ,  \"τ1\" -> 0.014453445820   ,  \"τS\" -> 0.020307523387   ,  \"τN\" -> 0.000603631080   ,  \"τC\" -> 0.003979837118   ,  \"κ0\" -> 0.000000005461   ,  \"mm1\" -> 0.000067516424   ,  \"mm2\" -> 0.013684499465   ,  \"mm3\" -> 0.026022826375   ,  \"T\" -> 0.830000000000   ,  \"B\" -> 12.000000000000   ,  \"θ\" -> 45.000000000000   ,  \"Reoff\" -> -285714.285714287310   ,  \"Imoff\" -> 0.000000000000   ,  \"στ1\" -> 0.000994587731   ,  \"στS\" -> 0.000123451502   ,  \"στN\" -> 0.000021982366    |>   , \n\"IDS0320_210901_RAW_cal__sam_\" ->   <|    \"ζ\" -> 0.023591124045   ,  \"τ1\" -> 0.014910006225   ,  \"τS\" -> 0.019342950404   ,  \"τN\" -> 0.000752972387   ,  \"τC\" -> 0.004900413232   ,  \"κ0\" -> 0.000000005453   ,  \"mm1\" -> 0.000090864236   ,  \"mm2\" -> 0.013909604856   ,  \"mm3\" -> 0.026379958563   ,  \"T\" -> 0.830000000000   ,  \"B\" -> 12.000000000000   ,  \"θ\" -> 45.000000000000   ,  \"Reoff\" -> 0.000000000000   ,  \"Imoff\" -> 0.000000000000   ,  \"στ1\" -> 0.000000000000   ,  \"στS\" -> 0.000000000000   ,  \"στN\" -> 0.000000000000    |>   , \n\"IDS0321_210901_RAW_cal__ref_\" ->   <|    \"ζ\" -> 0.020614746765   ,  \"τ1\" -> 0.013682065369   ,  \"τS\" -> 0.016105139108   ,  \"τN\" -> 0.000397734649   ,  \"τC\" -> 0.005005824303   ,  \"κ0\" -> 0.000000007592   ,  \"mm1\" -> 0.000077785268   ,  \"mm2\" -> 0.013046561126   ,  \"mm3\" -> 0.022406619598   ,  \"T\" -> 1.130000000000   ,  \"B\" -> 12.000000000000   ,  \"θ\" -> 45.000000000000   ,  \"Reoff\" -> 0.000000000000   ,  \"Imoff\" -> 0.000000000000   ,  \"στ1\" -> 0.000000000000   ,  \"στS\" -> 0.000000000000   ,  \"στN\" -> 0.000000000000    |>   , \n\"IDS0321_210901_RAW_cal__sam_\" ->   <|    \"ζ\" -> 0.020215154826   ,  \"τ1\" -> 0.014105227254   ,  \"τS\" -> 0.015660924043   ,  \"τN\" -> 0.000525137036   ,  \"τC\" -> 0.005447728357   ,  \"κ0\" -> 0.000000007594   ,  \"mm1\" -> 0.000080798630   ,  \"mm2\" -> 0.013233003317   ,  \"m
